vi "Clear Queues.vi"(8 "error in (no error)":errorcluster, 11 "Work Dispatcher in":refnum<class "Work Dispatcher.lvclass">) -> (0 "error out":errorcluster, 3 "Work Dispatcher out":refnum<class "Work Dispatcher.lvclass">)   [LabVIEW 2020, in "Work Dispatcher.lvclass"]
uses:
  Work Dispatcher.lvclass
  People/Process Job/Job Handler.lvclass
  Work Dispatcher.lvclass/Work Dispatcher.ctl
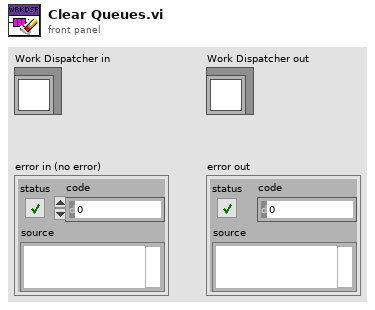
[diagram p1: front panel]
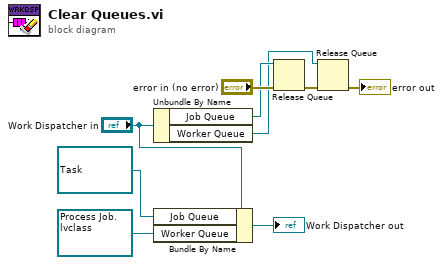
[diagram p0: block diagram]
diagram:
  n1 = Unbundle By Name("Work Dispatcher in") -> ("Job Queue"=w5:refnum<queue>, "Worker Queue"=w4:refnum<queue>)
  n2 = Bundle By Name(cluster="Work Dispatcher in", "Job Queue"=refnum<queue> refnum ("Task Queue"), "Worker Queue"=refnum<queue> refnum) -> (→"Work Dispatcher out":refnum<class "Work Dispatcher.lvclass">)
  n3 = Release Queue(queue=w5, error in (no error)="error in (no error)") -> (error out=w7:errorcluster)  [unwired: 1 in, 2 out]
  n4 = Release Queue(queue=w4, error in (no error)=w7) -> (error out=→"error out":errorcluster)  [unwired: 1 in, 2 out]
